vi "Configure Channel (Volt Normal).vi"(0 "VISA resource name":refnum<visa-resource-name>, 5 "Channel (0001)":string="0001", 7 "Enable Channel (True)":bool=TRUE, 9 "Range And Span":T1={"Volt Range (4 : 2V)"=4, "Enable Span (False)"=FALSE, "Lower Span (-2.0000)"=-2.0, "Upper Span (2.0000)"=2.0, "Bias (0)"=0.0} {"Upper Span (2.0000)" min=-99999.0 max=99999.0 step=1.0 format="%_5g"; "Lower Span (-2.0000)" min=-99999.0 max=99999.0 step=1.0 format="%_5g"; "Volt Range (4 : 2V)" items=["20mV", "60mV", "200mV", "1V", "2V", "6V", "20V", "50V"]}, 11 "error in (no error)":errorcluster) -> (4 "VISA resource name out":refnum<visa-resource-name>, 6 "Channel":string, 15 "error out":errorcluster)   [LabVIEW 2020, in "Yokogawa GX Series.lvlib"]
doc: "Sets the input range as voltage.\n\nCommand: SRangeAI"
uses:
  <instrlib>/Yokogawa GX Series/Yokogawa GX Series.lvlib
  <instrlib>/Yokogawa GX Series/Private/Volt Range.vi
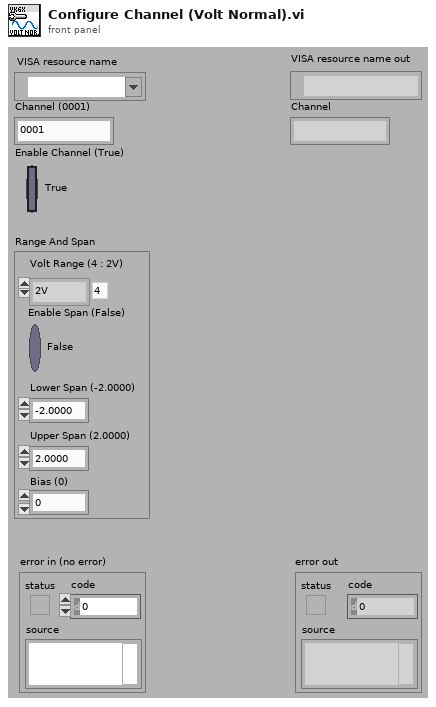
[diagram p1: front panel]
types:
  T1 = cluster{"Volt Range (4 : 2V)":i32, "Enable Span (False)":bool, "Lower Span (-2.0000)":dbl, "Upper Span (2.0000)":dbl, "Bias (0)":dbl}
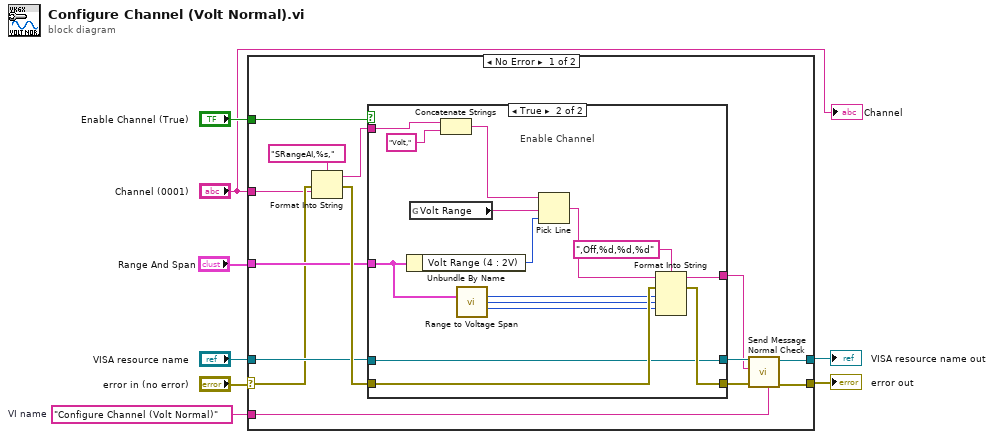
[diagram p0: block diagram]
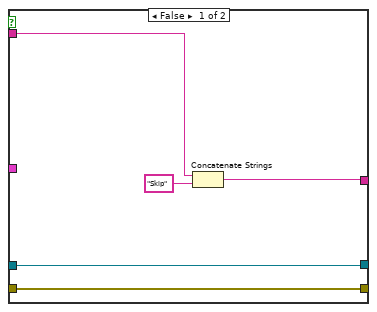
[diagram p2: hidden frame]
diagram:
  w4 = "Configure Channel (Volt Normal)"  # VI name
  n1 = case shown="No Error" "error in (no error)" {
    selector: "error in (no error)" -> [w10 w43]
    tunnel: "Enable Channel (True)" -> [w19 _]
    tunnel: "VISA resource name" -> [w18 w44]
    tunnel: [w15 w44] -> w6
    tunnel: [w14 w43] -> w5
    tunnel: w4 -> [w13 _]
    tunnel: "Range And Span" -> [w11 _]
    tunnel: "Channel (0001)" -> [w9 _]
    frame No Error {
      n2 = Format Into String(format string="SRangeAI,%s,", error in=w10, w9) -> (resulting string=w20:string, error out=w21:errorcluster)  [unwired: 1 in]
      n3 = case shown="True" w19 {
        tunnel: w21 -> [w24 w35]
        tunnel: [w24 w41] -> w16
        tunnel: w20 -> [w25 w39]
        tunnel: [w27 w38] -> w12
        tunnel: w18 -> [w23 w30]
        tunnel: [w23 w30] -> w17
        tunnel: w11 -> [_ w31]
        frame False {
          n4 = Concatenate Strings(w25, "Skip") -> (w27:string)
        }
        frame True {
          # "Enable Channel"
          n5 = Unbundle By Name(w31) -> ("Volt Range (4 : 2V)"=w32:i32)
          n6 = global read "Volt Range.vi" "Volt Range"() -> (w28:string)
          n7 = Concatenate Strings(w39, "Volt,") -> (w37:string)
          n8 = call <instrlib>:"Range to Voltage Span.vi"("Range And Span"=w31) -> ("Lower Span"=w29:i32, "Upper Span"=w34:i32, "Bias"=w33:i32)  [unwired: 7 in, 5 out]
          n9 = Pick Line(string ("")=w37, multi-line string=w28, line index=w32) -> (output string=w40:string)
          n10 = Format Into String(format string=",Off,%d,%d,%d", initial string=w40, error in=w35, w29, w34, w33) -> (resulting string=w38:string, error out=w41:errorcluster)
        }
      }
      n11 = call <instrlib>:"Send Message Normal Check.vi"("Source (\"\")"=w13, "error in (no error)"=w16, "Send Message (\"\")"=w12, "VISA resource name"=w17) -> ("error out"=w14:errorcluster, "VISA resource name out"=w15:refnum<visa-resource-name>)  [unwired: 2 in, 4 out]
    }
    frame Error {
    }
  }
  "error out" <- w5
  "VISA resource name out" <- w6
  "Channel" <- "Channel (0001)"
